vi "Reset Pins.vi"(8 "error in (no error)":errorcluster, 9 "Chip Address (A2 A1 A0)":T1 max=7, 10 "Slot #":T2 max=15, 11 "Rack #":u8) -> (0 "error out":errorcluster, 3 "SPI FIFO Message":u64)   [LabVIEW 2014, in "SLSC configuration Shared.lvlib"]
doc: "Configures the DIO board (IOCON.BANK = 0 - sequential addressing, switch all pins to outputs)."
uses:
  SLSC configuration Shared.lvlib
  Slot #.ctl
  MCP23S17/Chip Address.ctl
  MCP23S17/Write Digital All Pins.vi
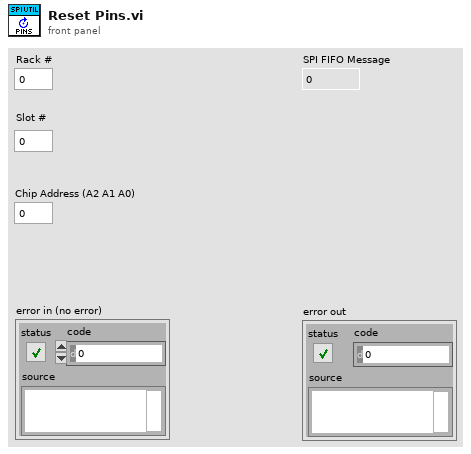
[diagram p1: front panel]
types:
  T1 = typedef "SLSC configuration Shared.lvlib/Chip Address.ctl" = u8
  T2 = typedef "SLSC configuration Shared.lvlib/Slot #.ctl" = u8
  T3 = typedef "SLSC configuration Shared.lvlib/SPI Command.ctl" = cluster{"SPI Command":u32, "Transfer Length":u8}
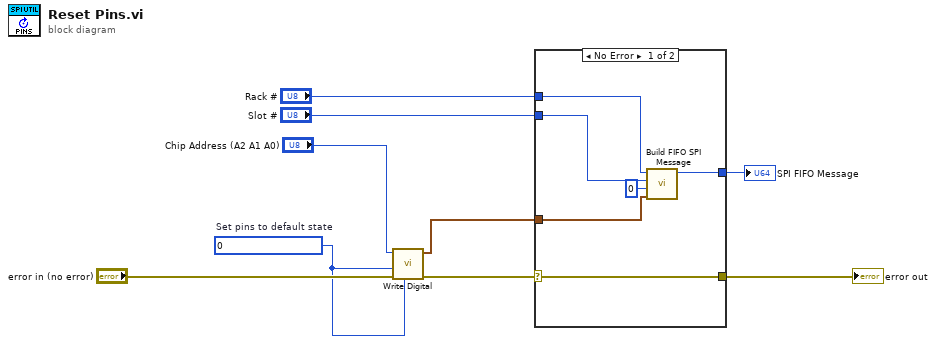
[diagram p0: block diagram]
diagram:
  w3 = u16 0  # Set pins to default state
  n1 = call-poly "Write Digital.vi"("Output Cache in"=w3, "error in (no error)"="error in (no error)", "Value"=w3, "Chip Address (A2 A1 A0)"="Chip Address (A2 A1 A0)") -> ("error out"=w5:errorcluster, "SPI Command"=w4:T3)  [unwired: 5 in, 1 out]
  n2 = case shown="No Error" w5 {
    selector: w5 -> [w13 w16]
    tunnel: w4 -> [w15 _]
    tunnel: [w14 _] -> w1
    tunnel: [w13 w16] -> w8
    tunnel: "Slot #" -> [w12 _]
    tunnel: "Rack #" -> [w11 _]
    frame No Error {
      n3 = call "Build FIFO SPI Message.vi"("SPI Command"=w15, "Chip Select"=u8 0, "Slot #"=w12, "Rack #"=w11) -> ("FIFO SPI Message"=w14:u64)  [unwired: 7 in]
    }
    frame Error {
    }
  }
  "error out" <- w8
  "SPI FIFO Message" <- w1
